vi "Double to Word.vi"(0 "Word":T1 {"Param Setting"."Num Bits" min=1 max=32; "Param Setting"."Start Bit" min=8 max=31; "Block Data Refs"."Data Reference" format="%.0x"}, 7 "Doubles In []":dbl[](array[numeric]), 11 "Channel FIFO Buffer Index":i32[](array[numeric])) -> (8 "Word":u32)   [LabVIEW 2017, in "Ballard Arinc-429 Engine.lvlib"]
uses:
  RT Driver/Ballard Arinc-429 Engine.lvlib
  RT Driver/RT Controls/RT Word Settings.ctl
  <vilib>/NI Veristand/Custom Device API/Block Data Reference.ctl
  <vilib>/NI Veristand/Custom Device API/Data Reference.ctl
  RT Driver/RT Controls/RT Param Setting.ctl
  Controls and Global/Start Bit.ctl
  Controls and Global/Number of Bits.ctl
  Ballard Arinc-429 Shared.lvlib
  <vilib>/NI Veristand/Custom Device API/Custom Device API.lvlib
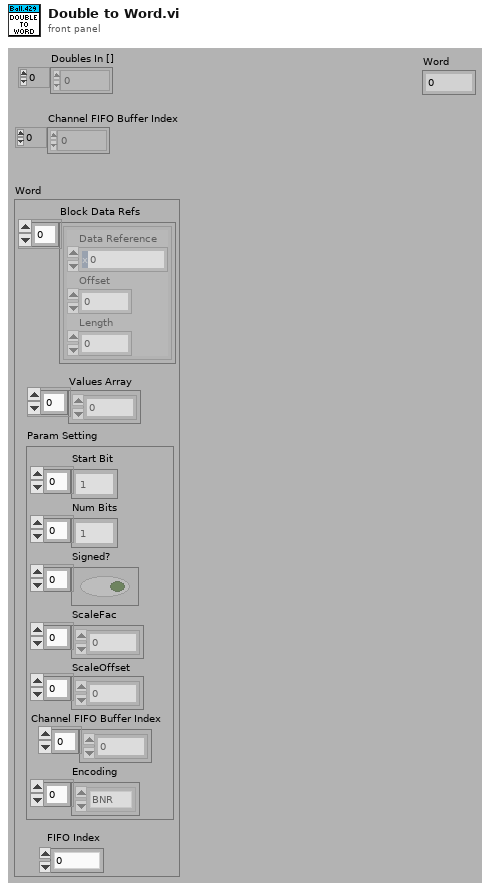
[diagram p1: front panel]
types:
  T1 = typedef "Ballard Arinc-429 Engine.lvlib/RT Word Settings.ctl" = cluster{"Block Data Refs":T2[], "Values Array":dbl[], "Length":i32, "FIFO Index":i32, "Param Setting":T4}
  T2 = typedef "Custom Device API.lvlib/Block Data Reference.ctl" = cluster{"Data Reference":T3, "Offset":u64, "Length":u64}
  T3 = typedef "Custom Device API.lvlib/Data Reference.ctl" = i32
  T4 = typedef "Ballard Arinc-429 Engine.lvlib/RT Param Setting.ctl" = cluster{"Start Bit":T5[], "Num Bits":T6[], "Signed?":bool[], "ScaleFac":dbl[], "ScaleOffset":dbl[], "Channel FIFO Buffer Index":i32[], "Encoding":enum16{"BNR", "BCD", "Discrete"}[]}
  T5 = typedef "Ballard Arinc-429 Shared.lvlib/Start Bit.ctl" = i32
  T6 = typedef "Ballard Arinc-429 Shared.lvlib/Number of Bits.ctl" = i32
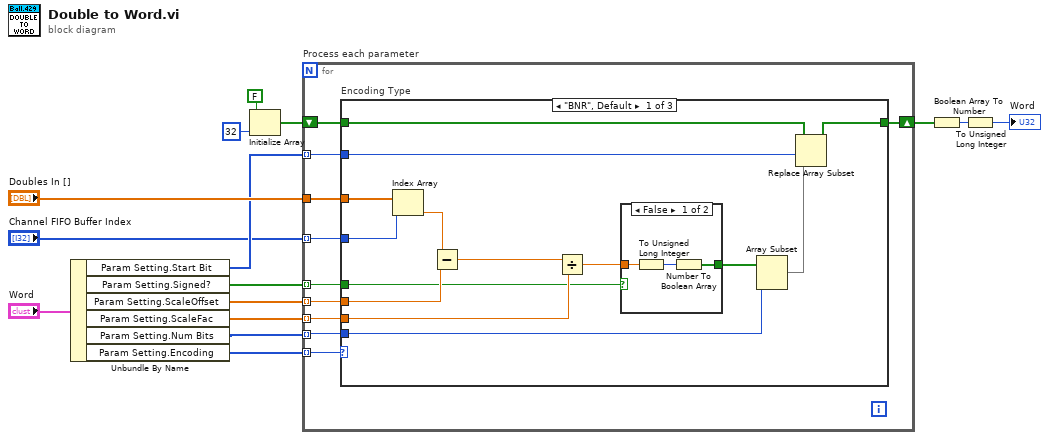
[diagram p0: block diagram]
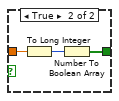
[diagram p2: hidden frame]
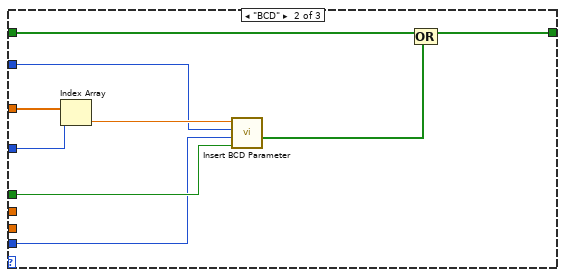
[diagram p3: hidden frame]
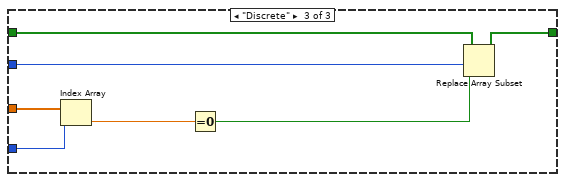
[diagram p4: hidden frame]
diagram:
  n1 = Unbundle By Name("Word") -> ("Param Setting.Start Bit"=w4:T5[], "Param Setting.Signed?"=w3:bool[], "Param Setting.ScaleOffset"=w14:dbl[], "Param Setting.ScaleFac"=w11:dbl[], "Param Setting.Num Bits"=w13:T6[], "Param Setting.Encoding"=w1:enum16{"BNR", "BCD", "Discrete"}[])
  n2 = Initialize Array(FALSE, 32 ("dimension size")) -> (w10:bool[])
  n3 = for "Process each parameter" {
    tunnel: w11 -> [w25] mode=indexing
    shift-right: [w24] -> w7
    shift-left: w10 -> [w23]
    tunnel: w4 -> [w22] mode=indexing
    tunnel: w14 -> [w21] mode=indexing
    tunnel: w13 -> [w20] mode=indexing
    tunnel: "Doubles In []" -> [w18]
    tunnel: w3 -> [w19] mode=indexing
    tunnel: "Channel FIFO Buffer Index" -> [w17] mode=indexing
    tunnel: w1 -> [w16] mode=indexing
    n4 = case "Encoding Type" shown="\"BNR\", Default" w16 {
      tunnel: w25 -> [w38 _ _]
      tunnel: [w34 w51 w61] -> w24
      tunnel: w23 -> [w33 w52 w60]
      tunnel: w22 -> [w26 w47 w59]
      tunnel: w21 -> [w32 _ _]
      tunnel: w20 -> [w31 w46 _]
      tunnel: w19 -> [w30 w49 _]
      tunnel: w18 -> [w29 w54 w58]
      tunnel: w17 -> [w28 w53 w57]
      frame "BNR", Default {
        n5 = Index Array(array=w29, index=w28) -> (element=w27:dbl)
        n6 = Subtract(x=w27, y=w32) -> (x-y=w39:dbl)
        n7 = Divide(x=w39, y=w38) -> (x/y=w37:dbl)
        n8 = case shown="False" w30 {
          tunnel: w37 -> [w42 w45]
          tunnel: [w40 w43] -> w36
          frame False {
            n9 = To Unsigned Long Integer(number=w42) -> (unsigned 32bit integer=w41:u32)
            n10 = Number To Boolean Array(number=w41) -> (Boolean array=w40:bool[])
          }
          frame True {
            n11 = To Long Integer(number=w45) -> (32bit integer=w44:i32)
            n12 = Number To Boolean Array(number=w44) -> (Boolean array=w43:bool[])
          }
        }
        n13 = Array Subset(array=w36, length=w31) -> (w35:bool[])  [unwired: 1 in]
        n14 = Replace Array Subset(array=w33, new element=w35, index=w26) -> (w34:bool[])
      }
      frame "BCD" {
        n15 = Index Array(array=w54, index=w53) -> (element=w50:dbl)
        n16 = call "Insert BCD Parameter.vi"("Signed?"=w49, "Number of Bits"=w46, "Start Bit"=w47, "BCD Value"=w50) -> ("BCD Mask"=w48:bool[])  [unwired: 6 in, 1 out]
        n17 = Compound Arithmetic op=OR(w52, w48) -> (w51:bool[])
      }
      frame "Discrete" {
        n18 = Index Array(array=w58, index=w57) -> (element=w56:dbl)
        n19 = Equal To 0?(x=w56) -> (x = 0?=w55:bool)
        n20 = Replace Array Subset(array=w60, new element=w55, index=w59) -> (w61:bool[])
      }
    }
  }
  n21 = Boolean Array To Number(Boolean array=w7) -> (number=w6:u32)
  n22 = To Unsigned Long Integer(number=w6) -> (unsigned 32bit integer=→"Word":u32)
